vi "firmware_version.vi"() -> ()   [LabVIEW 2020]
panel:
  out "Terminal Output":string
  in  "Python Fucntion Path":path=path "C:/Users/emily/Documents/zedboard/examples-git"
  out "Error Out":errorcluster
  in  "FMC Parameters":T1={"IP"="192.168.1.193", "Port"=22, "Username"="analog", "Password"="analog"}
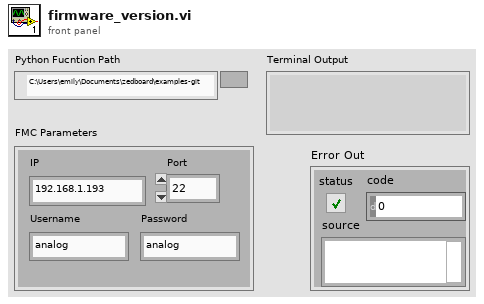
[diagram p1: front panel]
types:
  T1 = cluster{"IP":string, "Port":i32, "Username":string, "Password":string}
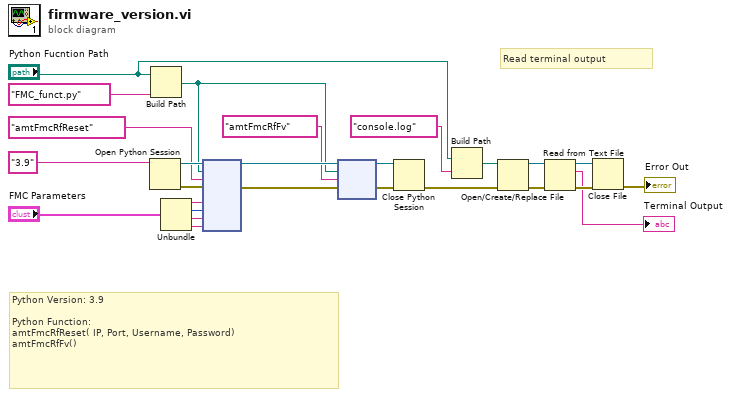
[diagram p0: block diagram]
diagram:
  # "Read terminal output"
  # "Python Version: 3.9\n\nPython Function:\namtFmcRfReset( IP, Port, Username, Password)\namtFmcRfFv()"
  n1 = Open Python Session(python version="3.9" ("Python version")) -> (session out=w20:refnum<k35>, error out=w21:errorcluster)  [unwired: 2 in]
  n2 = Build Path(base path="Python Fucntion Path", name or relative path="FMC_funct.py") -> (appended path=w13:path)
  n3 = Unbundle("FMC Parameters") -> ("IP"=w25:string, "Port"=w24:i32, "Username"=w23:string, "Password"=w22:string)
  n4 = node(w20, w13, "amtFmcRfReset" ("function name"), w21, w25, w24, w23, w22) -> (w16:refnum<k35>, w15:errorcluster)  [unwired: 6 in, 2 out]
  n5 = node(w16, w13, "amtFmcRfFv" ("function name"), w15) -> (w3:refnum<k35>, w4:errorcluster)  [unwired: 2 in, 2 out]
  n6 = Close Python Session(session in=w3, error in=w4) -> (11:w6:errorcluster)
  n7 = Build Path(base path="Python Fucntion Path", name or relative path="console.log" ("function name")) -> (appended path=w12:path)
  n8 = Open/Create/Replace File(file path (use dialog)=w12, error in=w6) -> (refnum out=w7:refnum<file>, error out=w10:errorcluster)  [unwired: 4 in, 1 out]
  n9 = Read from Text File(file (use dialog)=w7, error in=w10) -> (refnum out=w8:refnum<file>, text=→"Terminal Output":string, error out=w9:errorcluster)  [unwired: 2 in, 1 out]
  n10 = Close File(refnum=w8, error in=w9) -> (error out=→"Error Out":errorcluster)  [unwired: 1 out]
